vi "Test List Parametrized Test Cases Second Parameter.vi"(11 "Test Case In":refnum<class "Parameterized Test Case Test.lvclass">) -> (0 "error out":errorcluster, 3 "Test Case Out":refnum<class "Parameterized Test Case Test.lvclass">)   [LabVIEW 2020, in "Parameterized Test Case Test.lvclass"]
uses:
  Parameterized Test Case Test.lvclass
  C:/Program Files (x86)/National Instruments/LabVIEW 2020/vi.lib/Astemes/LUnit/Test Case.lvclass
  source/Parametrized Test Case Test Double/Parametrized Test Case Test Double.lvclass
  <vilib>/Astemes/LUnit/Test Case.lvclass/Test Case.ctl
  399136ac-e113-4bca-be3a-8dde4e32c814.vi
  <vilib>/Astemes/LUnit/Palette/Pass If.vi
  <vilib>/Astemes/LUnit/Append Fail Result.vi
  <vilib>/Astemes/LUnit/Append Pass Result.vi
  <vilib>/Astemes/LUnit/Run In UI.vi
  <vilib>/Utility/error.llb/Clear Errors.vi
  Parameterized Test Case Test.lvclass/Parameterized Test Case Test.ctl
  <vilib>/Astemes/LUnit/Test Suite.lvclass
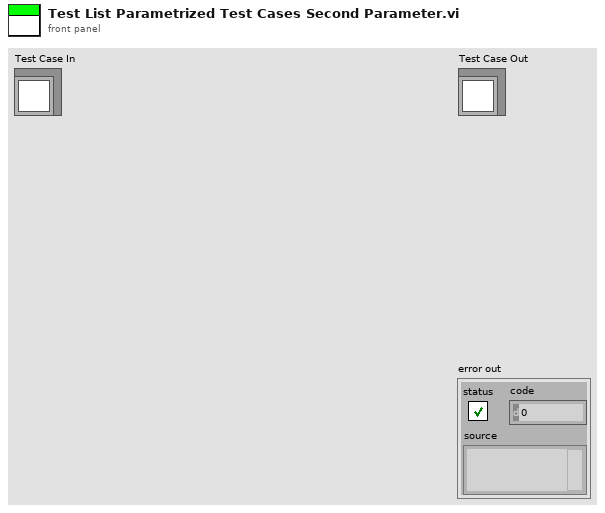
[diagram p1: front panel]
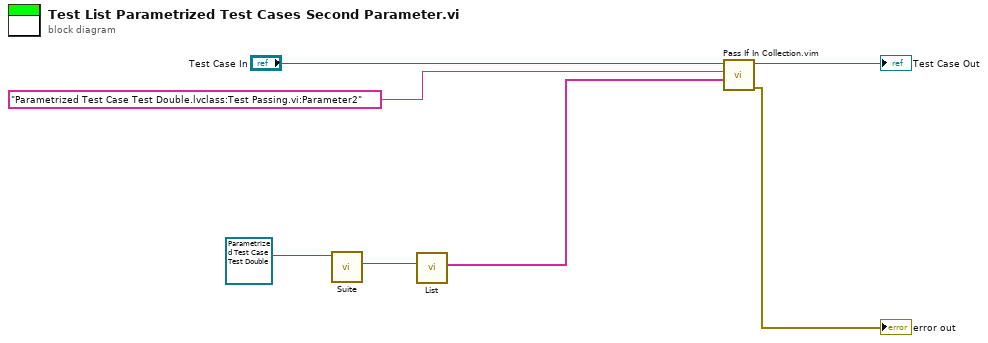
[diagram p0: block diagram]
diagram:
  n1 = call-dynamic "Suite.vi"("Parameterized Test Case In"=refnum<class "Parametrized Test Case Test Double.lvclass"> refnum ("Parametrized Test Case Test Double.lvclass")) -> ("LUnit Test Suite Out"=w2:refnum<class "Test Suite.lvclass">)  [unwired: 8 in, 2 out]
  n2 = call <vilib>:"List.vi"("LUnit Test Suite In"=w2) -> ("List of Runnables"=w1:string[])  [unwired: 9 in, 1 out]
  n3 = call "Pass If In Collection.vim"("Collection"=w1, "Expected Element"="Parametrized Test Case Test Double.lvclass:Test Passing.vi:Parameter2" ("String"), "LUnit Test Case In"="Test Case In") -> ("error out"=→"error out":errorcluster, "LUnit Test Case Out"=→"Test Case Out":refnum<class "Parameterized Test Case Test.lvclass">)  [unwired: 7 in]
